vi "Controller Module.vi"(8 "error in":errorcluster) -> (0 "error out":errorcluster)   [LabVIEW 2018, in "Controller.lvlib"]
doc: "This is the top level of the controller module (a free running module of the Car WAsh simulator). The client must be stipulated by either the launcher or the controller.\n\nIt is closed using a user event. It communicates with the other modules using a queue based API which has comms modules that can be swapped if required."
uses:
  Controller.lvlib
  Entry Console/Entry Console/Public Controls/Entry Console.ctl
  Private Controls/Module Data Cluster.ctl
  Private Controls/Module Action.ctl
  <vilib>/Utility/error.llb/DialogType.ctl
  User Events/controls/Actions.ctl
  Display Console/Display Console/public controls/Display Data.ctl
  Entry Console/Entry Console/Public Controls/Button Status.ctl
  Display Console/Display Console/Display.lvlib
  Entry Console/Entry Console/Entry Console.lvlib
  Database/Database.lvlib
panel:
  in  "client":string
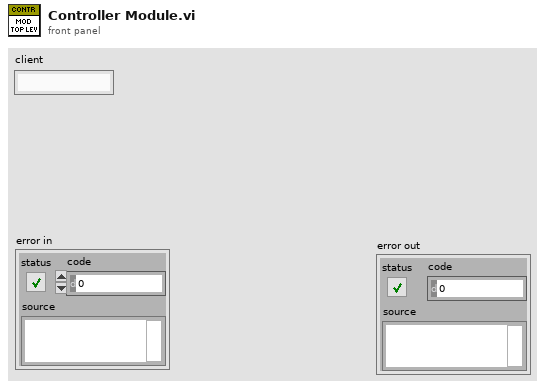
[diagram p1: front panel]
types:
  T1 = cluster{"Step Duration":string, "Station":string, "Wash Step":string}[]
  T2 = typedef "Entry Console.lvlib/Entry Console.ctl" = cluster{"Variant":variant}
  T3 = typedef "Actions.ctl" = enum16{"Get", "Create", "Destroy"}
  T4 = typedef "Display.lvlib/Display Data.ctl" = cluster{"Variant":variant}
  T5 = typedef "Controller.lvlib/Module Data Cluster.ctl" = cluster{"Variant":variant, "action":T6}
  T6 = typedef "Controller.lvlib/Module Action.ctl" = enum16{"error", "exit", "init", "start", "Action", "Receive Config Data"}
  T7 = cluster{"Variant":variant, "action":enum16{"error", "exit", "init"}}
  T8 = typedef "DialogType.ctl" = u16
  T9 = typedef "Entry Console.lvlib/Button Status.ctl" = cluster{"Enable  ctrl1":bool, "reset":bool, "Enable ctrl2":bool}
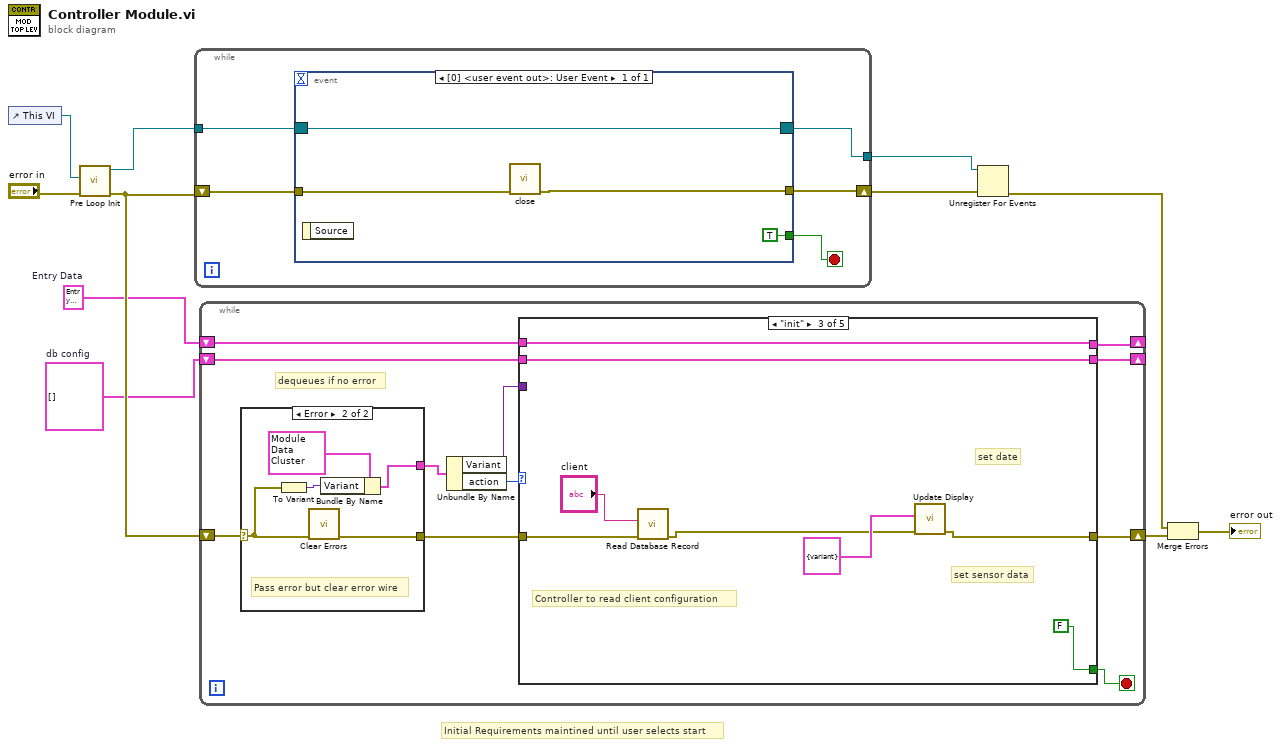
[diagram p0: block diagram]
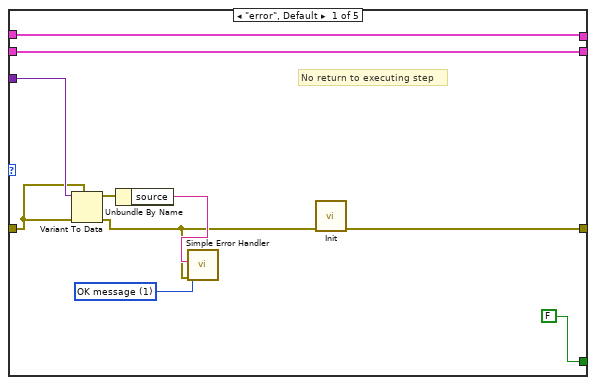
[diagram p2: hidden frame]
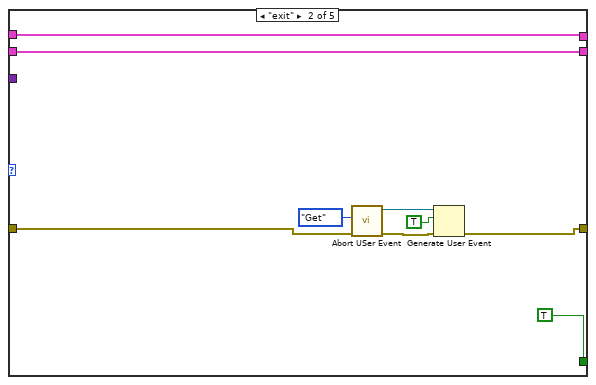
[diagram p3: hidden frame]
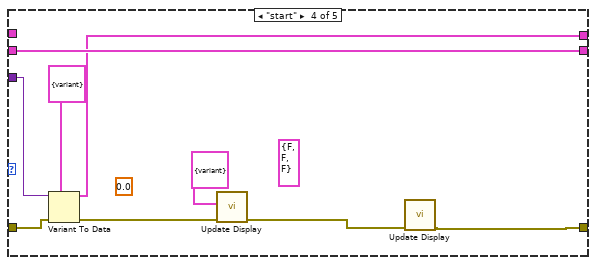
[diagram p4: hidden frame]
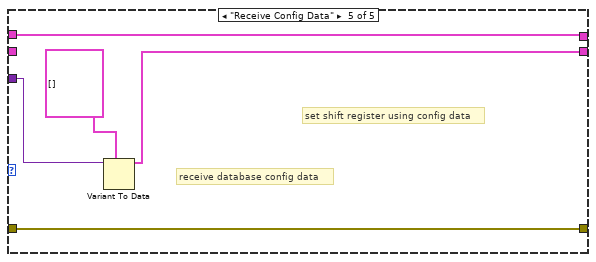
[diagram p5: hidden frame]
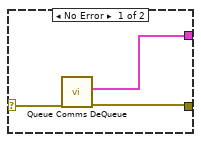
[diagram p6: hidden frame]
diagram:
  w1 = T1 []  # db config
  w2 = T2 {"Variant"=variant}  # Entry Data
  # "Initial Requirements maintined until user selects start"
  n1 = control-ref of="This VI"() -> (w11:refnum<vi>)
  n2 = call "Pre Loop Init.vi"("error in"="error in", "Ref In"=w11) -> ("error out"=w8:errorcluster, "Event Registration Refnum"=w10:refnum<event-registration>)  [unwired: 8 in]
  n3 = while {
    shift-right: [w15] -> w7
    shift-left: w8 -> [w16]
    tunnel: w10 -> [w14]
    tunnel: [w12] -> w6
    stop <- w13 stop-if-true
    n4 = event shown="[0] <user event out>: User Event" {
      selector: w14 -> [w17]
      dyn-events: [w17] -> w12
      timeout: _ -> [_]
      tunnel: w16 -> [w20]
      tunnel: [w19] -> w15
      tunnel: [TRUE] -> w13
      event User Event {
        n5 = event-data() -> ()  [unwired: 1 in, 1 out]
        n6 = call "close.vi"("error in"=w20) -> ("error out"=w19:errorcluster)  [unwired: 10 in]
      }
    }
  }
  n7 = while {
    shift-right: [w27] -> w5
    shift-left: w8 -> [w31]
    shift-right: [w24] -> _
    shift-left: w1 -> [w23]
    shift-right: [w22] -> _
    shift-left: w2 -> [w21]
    stop <- w25 stop-if-true
    # "dequeues if no error"
    n8 = case shown="Error" w31 {
      selector: w31 -> [w75 w80]
      tunnel: [w74 w76] -> w30
      tunnel: [w73 w79] -> w26
      frame No Error {
        n9 = call "Queue Comms DeQueue.vi"("error in"=w75) -> ("error out"=w73:errorcluster, "element"=w74:T7)  [unwired: 9 in]
      }
      frame Error {
        # "Pass error but clear error wire"
        n10 = To Variant(anything=w80) -> (Variant=w77:variant)
        n11 = call <vilib>:"Clear Errors.vi"("error in (no error)"=w80) -> ("error out"=w79:errorcluster)  [unwired: 5 in, 1 out]
        n12 = Bundle By Name(cluster=T5 {"Variant"=variant, "action"=enum."error"} ("element"), "Variant"=w77) -> (w76:T5)
      }
    }
    n13 = Unbundle By Name(w30) -> ("Variant"=w28:variant, "action"=w29:T6)
    n14 = case shown="\"init\"" w29 {
      tunnel: w28 -> [w37 _ _ w65 w71]
      tunnel: [w33 w42 w51 w61 w72] -> w27
      tunnel: w26 -> [w36 w43 w57 w63 w72]
      tunnel: [FALSE TRUE FALSE _ _] -> w25
      tunnel: [w40 w49 w54 w66 w70] -> w24
      tunnel: w23 -> [w40 w49 w54 w66 _]
      tunnel: [w39 w48 w53 w62 w69] -> w22
      tunnel: w21 -> [w39 w48 w53 _ w69]
      frame "error", Default {
        w38 = T8 1 items=["no dialog", "OK message", "continue or stop message", "OK message + warnings", "continue/stop + warnings"] ("type of dialog (OK msg:1)")
        # "No return to executing step"
        n15 = Variant To Data(error in=w36, type=w36, Variant=w37) -> (data=w35:errorcluster, error out=w32:errorcluster)
        n16 = Unbundle By Name(w35) -> ("source"=w34:string)
        n17 = call <vilib>:"Simple Error Handler.vi"("error source (\" \")"=w34, "type of dialog (OK msg:1)"=w38, "error in (no error)"=w32) -> ()  [unwired: 2 in, 5 out]
        n18 = call "Init.vi"("error in"=w32) -> ("error out"=w33:errorcluster)  [unwired: 10 in]
      }
      frame "exit" {
        n19 = call "Abort USer Event.vi"("error in"=w43, "Enum"=Actions."Get") -> ("error out"=w45:errorcluster, "user event out"=w44:refnum<user-event>)  [unwired: 8 in]
        n20 = Generate User Event(user event=w44, event data cluster=TRUE ("event data"), error in=w45) -> (error out=w42:errorcluster)  [unwired: 1 in, 1 out]
      }
      frame "init" {
        # "set sensor data"
        # "set date"
        # "Controller to read client configuration"
        n21 = call "Read Database Record.vi"("error in"=w57, "data"="client") -> ("error out"=w52:errorcluster)  [unwired: 9 in]
        n22 = call "Update Display.vi"("error in"=w52, "data"=T4 {"Variant"=variant(cluster{"Variant":variant} {"Variant"=variant})} ("Cluster")) -> ("error out"=w51:errorcluster)  [unwired: 9 in]
      }
      frame "start" {
        (unwired) 0.0
        (unwired) T9 {"Enable  ctrl1"=FALSE, "reset"=FALSE, "Enable ctrl2"=FALSE}
        n23 = Variant To Data(error in=w63, type=T2 {"Variant"=variant} ("WashStepSelection"), Variant=w65) -> (data=w62:T2, error out=w60:errorcluster)
        n24 = call "Update Display.vi"("error in"=w60, "data"=T4 {"Variant"=variant} ("Cluster")) -> ("error out"=w59:errorcluster)  [unwired: 9 in]
        n25 = call "Update Display.vi"("error in"=w59) -> ("error out"=w61:errorcluster)  [unwired: 10 in]
      }
      frame "Receive Config Data" {
        # "set shift register using config data"
        # "receive database config data"
        n26 = Variant To Data(type=T1 [], Variant=w71) -> (data=w70:T1)  [unwired: 1 in, 1 out]
      }
    }
  }
  n27 = Unregister For Events(event registration refnum=w6, error in=w7) -> (error out=w3:errorcluster)
  n28 = Merge Errors(w3, w5) -> (→"error out":errorcluster)
